vi "Cleanup (User).vi"(8 "error in":errorcluster, 11 "Node in":refnum<class "BLS Cycler Template.lvclass">) -> (0 "error in":errorcluster, 3 "Node out":refnum<class "BLS Cycler Template.lvclass">)   [LabVIEW 2023, in "BLS Cycler Template.lvlib" / "BLS Cycler Template.lvclass"]
uses:
  BLS Cycler Template.lvclass
  BLS Cycler Template.lvclass/BLS Cycler Template.ctl
  bls-capabilities/src/Capabilities/High Level Capabilities/Cycler/Cycler.lvclass
  bls-capabilities/src/Capabilities/High Level Capabilities/Cycler/Output Enable Write Single.vi
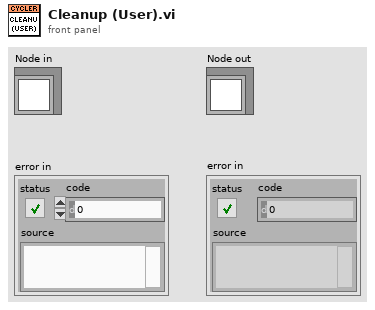
[diagram p1: front panel]
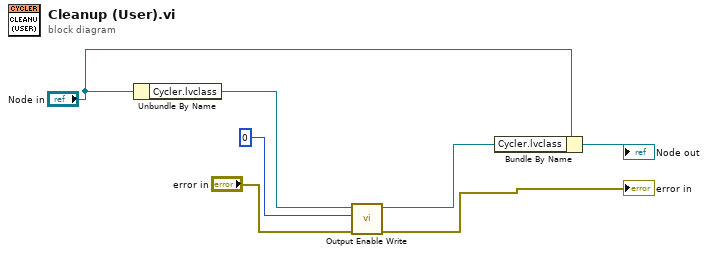
[diagram p0: block diagram]
diagram:
  n1 = Unbundle By Name("Node in") -> ("Cycler.lvclass"=w4:refnum<class "Cycler.lvclass">)
  n2 = call-poly "Output Enable Write.vi"("error in"="error in", "Output Enable STS"=0, "Cycler in"=w4) -> ("error out"=→"error in":errorcluster, "Cycler out"=w5:refnum<class "Cycler.lvclass">)  [unwired: 7 in]
  n3 = Bundle By Name(cluster="Node in", "Cycler.lvclass"=w5) -> (→"Node out":refnum<class "BLS Cycler Template.lvclass">)
